vi "line -- complex.vi"(8 "n":dbl, 10 "slope":cdb, 11 "intercept":cdb) -> (0 "value":cdb, 1 "tangent":cdb)   [LabVIEW 2015]
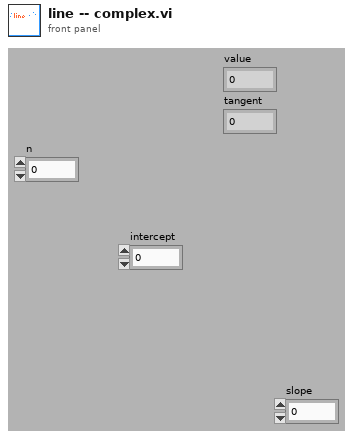
[diagram p1: front panel]
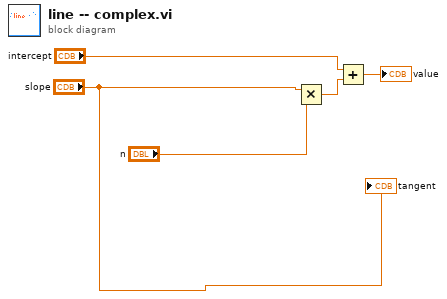
[diagram p0: block diagram]
diagram:
  n1 = Multiply(x="slope", y="n") -> (x*y=w5:cdb)
  n2 = Add(x="intercept", y=w5) -> (x+y=→"value":cdb)
  "tangent" <- "slope"
